vi "testQueueDll.vi"() -> ()   [LabVIEW 2011]
panel:
  out "元素":string
  in  "s":string
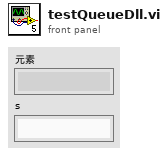
[diagram p1: front panel]
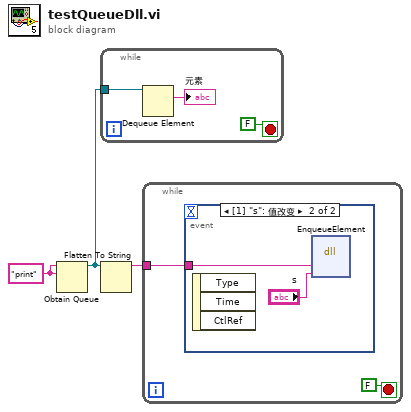
[diagram p0: block diagram]
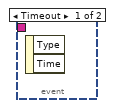
[diagram p2: hidden frame]
diagram:
  w2 = "print" ("queueName")
  n1 = Obtain Queue(name (unnamed)=w2, element data type=w2) -> (queue out=w1:refnum<queue>)  [unwired: 3 in, 2 out]
  n2 = while {
    tunnel: w1 -> [w5]
    stop <- FALSE stop-if-true
    n3 = Dequeue Element(queue=w5) -> (element=→"元素":string)  [unwired: 2 in, 3 out]
  }
  n4 = Flatten To String(anything=w1) -> (data string=w3:string)  [unwired: 3 in, 2 out]
  n5 = while {
    tunnel: w3 -> [w8]
    stop <- FALSE stop-if-true
    n6 = event shown="[1] \"s\": 值改变" {
      selector: _ -> [_ _]
      dyn-events: _ -> [_ _]
      timeout: _ -> [_ _]
      tunnel: w8 -> [_ w9]
      event Timeout {
        n7 = event-data() -> ()  [unwired: 1 in, 2 out]
      }
      event "s": Value Change {
        n8 = event-data() -> ()  [unwired: 1 in, 3 out]
        n9 = dll-call lib="PTH1Wabs GMy DBank\t_work_panLuaDllToLabviewbuilds\ttestC_dll\n我的DLL2\tqueue.dll" fn="EnqueueElement"("queue"=w9, "element"="s") -> ()  [unwired: 6 in, 2 out]
      }
    }
  }
